vi "Reset.vi"(0 "VISA resource name":refnum<visa-resource-name>, 11 "error in (no error)":errorcluster) -> (4 "VISA resource name out":refnum<visa-resource-name>, 15 "error out":errorcluster)   [LabVIEW 2014, in "Associated Power Technologies 8500 Series.lvlib"]
doc: "Reset the instrument to <B>original power on configuration</B>. Does not clear Enable register for Standard Summary Status or Standard Event Registers. Does not clear the output queue. Does not clear the power-on-status-clear flag."
uses:
  <instrlib>/Associated Power Technologies 8500 Series/Associated Power Technologies 8500 Series.lvlib
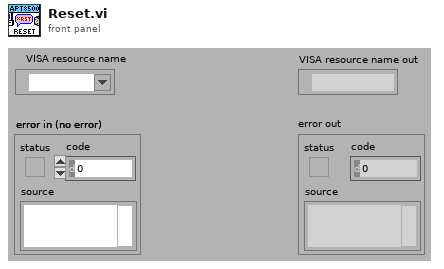
[diagram p1: front panel]
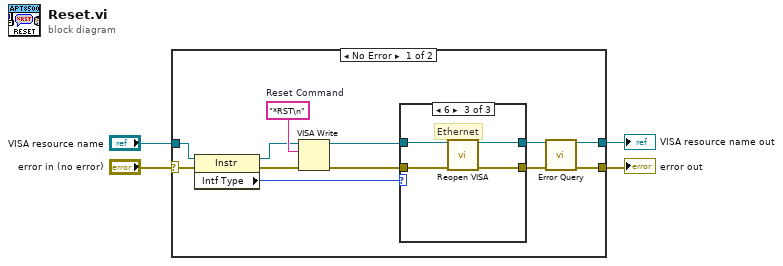
[diagram p0: block diagram]
diagram:
  n1 = case shown="No Error" "error in (no error)" {
    selector: "error in (no error)" -> [w13 w25]
    tunnel: "VISA resource name" -> [w12 w26]
    tunnel: [w16 w26] -> w3
    tunnel: [w15 w25] -> w2
    frame No Error {
      w14 = "*RST\n"  # Reset Command
      n2 = property on="Property Node" class="Instr"(reference=w12, error in=w13) -> (reference out=w11:refnum<visa-resource-name>, error out=w10:errorcluster, "Intf Type"=w9:u16)
      n3 = VISA Write(VISA resource name=w11, write buffer=w14, error in (no error)=w10) -> (VISA resource name out=w6:refnum<visa-resource-name>, error out=w5:errorcluster)  [unwired: 1 out]
      n4 = case shown="6" w9 {
        tunnel: w5 -> [w18 w20 w23]
        tunnel: [w18 w20 w22] -> w8
        tunnel: w6 -> [w17 w19 w24]
        tunnel: [w17 w19 w21] -> w7
        frame Default {
        }
        frame 1, 4 {
          # "GPIB. Serial"
        }
        frame 6 {
          # "Ethernet"
          n5 = call <instrlib>:"Reopen VISA.vi"("VISA resource name"=w24, "error in (no error)"=w23) -> ("VISA resource name out"=w21:refnum<visa-resource-name>, "error out"=w22:errorcluster)  [unwired: 12 in]
        }
      }
      n6 = call <instrlib>:"Error Query.vi"("VISA resource name"=w7, "error in (no error)"=w8) -> ("VISA resource name out"=w16:refnum<visa-resource-name>, "error out"=w15:errorcluster)  [unwired: 10 in, 2 out]
    }
    frame Error {
    }
  }
  "error out" <- w2
  "VISA resource name out" <- w3
